vi "SequenceEvent.PropertyChanged.vi"(4 "State":refnum<user-event>, 5 "Event Data":cluster{"sender":refnum<k24>, "e":refnum<k24>}, 6 "Control Ref":refnum<k24>, 7 "Event Common Data":T1) -> ()   [LabVIEW 2015, in "Single Station Execution.lvlib"]
uses:
  Single Station Execution.lvlib
  NationalInstruments.VeriStand.RealTimeSequenceDefinitionApi
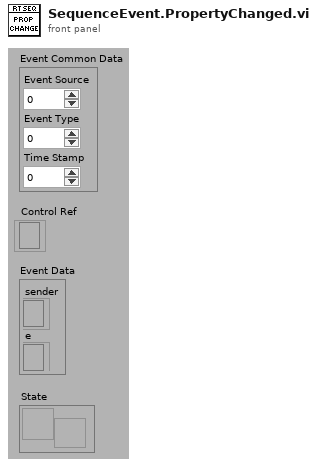
[diagram p1: front panel]
types:
  T1 = cluster{"Event Source":i32, "Event Type":u32, "Time Stamp":u32}
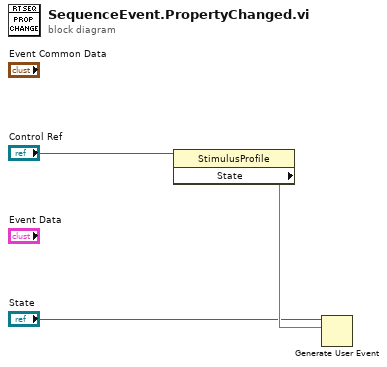
[diagram p0: block diagram]
diagram:
  n1 = property class="StimulusProfile"(reference="Control Ref") -> ("State"=w3)  [unwired: 1 in, 2 out]
  n2 = Generate User Event(user event="State", event data cluster=w3) -> ()  [unwired: 2 in, 2 out]
